vi "PI_ARW.vi"(3 "offset":dbl, 4 "Ti_value":dbl, 5 "p_value":dbl, 6 "Integrator enabled range":dbl, 7 "old error":dbl, 8 "actual error":dbl, 9 "ARW on/off":bool) -> (0 "new error":dbl, 2 "output":dbl)   [LabVIEW 2013]
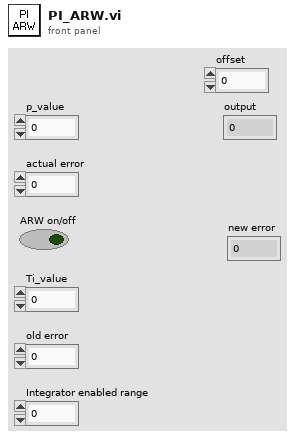
[diagram p1: front panel]
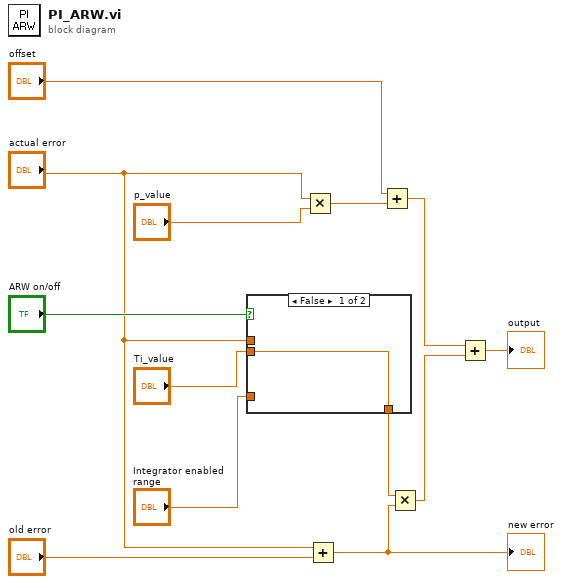
[diagram p0: block diagram]
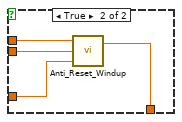
[diagram p2: hidden frame]
diagram:
  n1 = case shown="False" "ARW on/off" {
    tunnel: "Integrator enabled range" -> [_ w18]
    tunnel: [w14 w17] -> w7
    tunnel: "Ti_value" -> [w14 w16]
    tunnel: "actual error" -> [_ w15]
    frame False {
    }
    frame True {
      n2 = call "Anti_Reset_Windup.vi"("Integrator enabled range"=w18, "Ti_enabled_in"=w16, "actuall error"=w15) -> ("Ti_out"=w17:dbl)  [unwired: 1 in]
    }
  }
  n3 = Multiply(x="actual error", y="p_value") -> (x*y=w4:dbl)
  n4 = Add(x="actual error", y="old error") -> (x+y=w2:dbl)
  "new error" <- w2
  n5 = Add(x="offset", y=w4) -> (x+y=w5:dbl)
  n6 = Multiply(x=w7, y=w2) -> (x*y=w10:dbl)
  n7 = Add(x=w5, y=w10) -> (x+y=→"output":dbl)
